vi "GetImages.vi"(4 "File type":T1, 5 "Disabled":bool, 6 "Background Color":u32(colorbox), 7 "image directory":path, 8 "error in":errorcluster, 11 "Boolean in":refnum<class "Boolean.lvclass">) -> (0 "error out":errorcluster, 3 "Boolean out":refnum<class "Boolean.lvclass">)   [LabVIEW 2014, in "Raspberry Pi Compatible Compiler for LabVIEW.lvlib" / "Boolean.lvclass"]
uses:
  Boolean.lvclass
  Control/ImageTypes.ctl
  GObject/GObject.lvclass/GObject.ctl
  GObject/GObject.lvclass
  Raspberry Pi Compatible Compiler for LabVIEW.lvlib
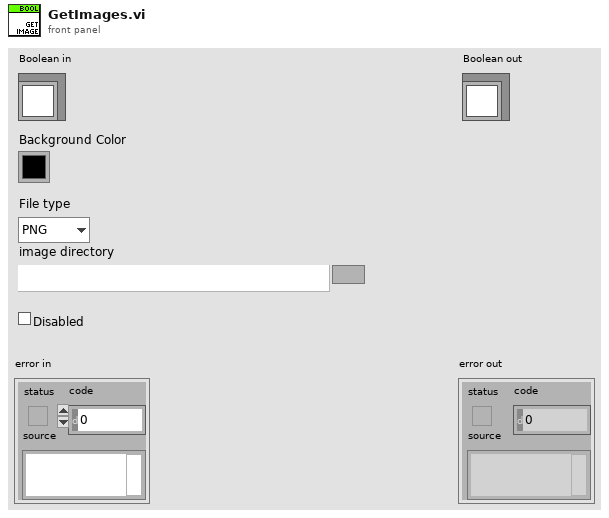
[diagram p1: front panel]
types:
  T1 = typedef "Raspberry Pi Compatible Compiler for LabVIEW.lvlib/ImageTypes.ctl" = enum16{"PNG", "JPEG", "BMP"}
  T2 = enum8{"Enabled", "Disabled", "Disabled and Grayed Out"}
  T3 = enum32{"Invalid", "Standard", "Closed", "Hidden", "Minimized", "Maximized"}
  T4 = typedef "LVPositionTypeDef.ctl" = cluster{"Left":i32, "Top":i32}
  T5 = typedef "imagedata.ctl" = cluster{"image type":i32, "image depth":i32, "image":u8[], "mask":u8[], "colors":u32[], "Rectangle":cluster{"left":i16, "top":i16, "right":i16, "bottom":i16}}
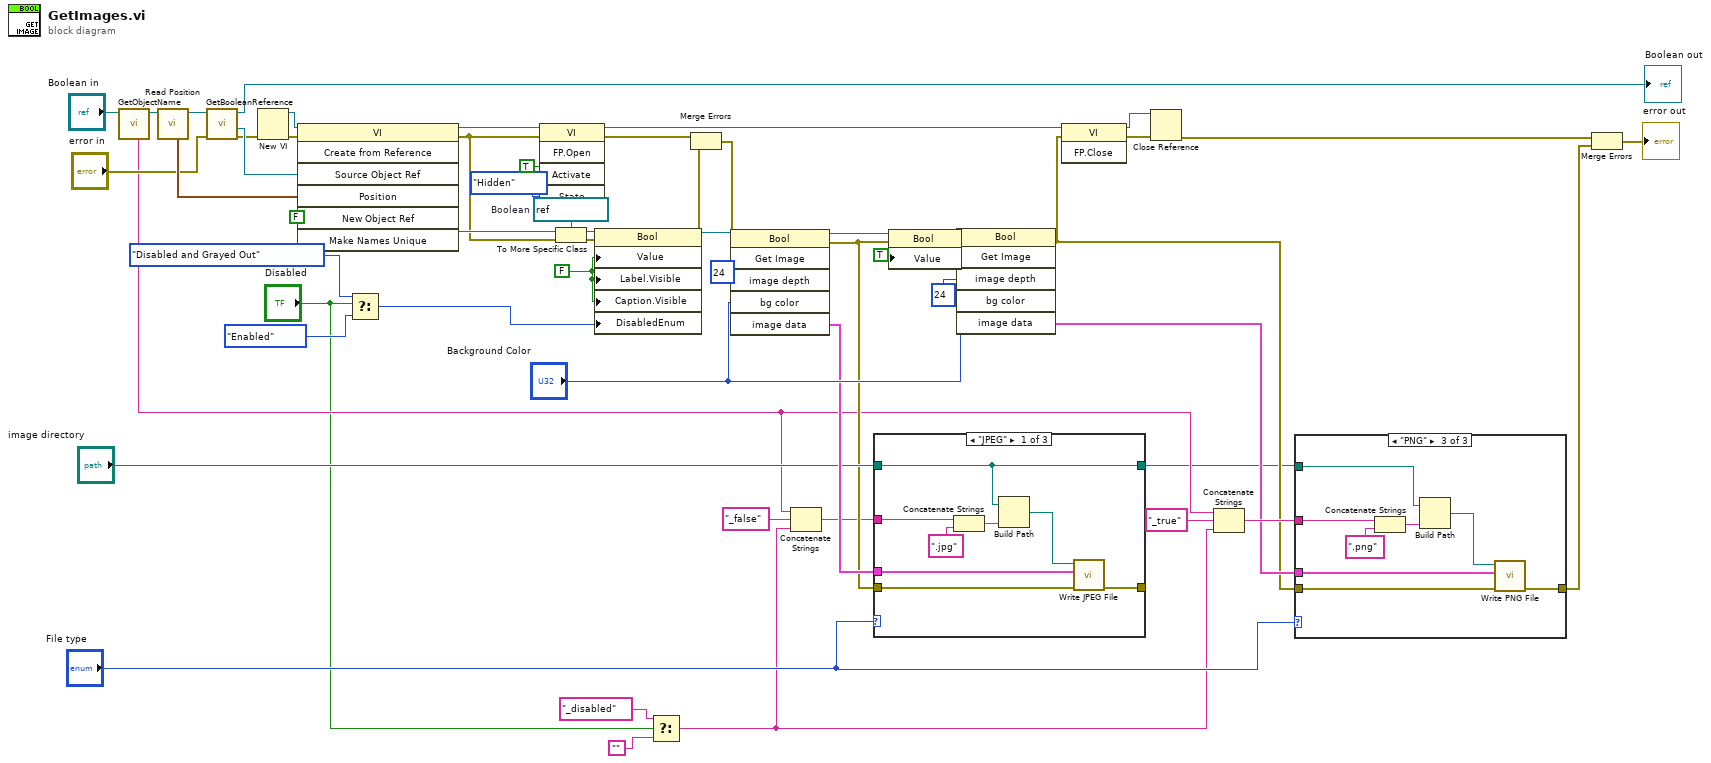
[diagram p0: block diagram]
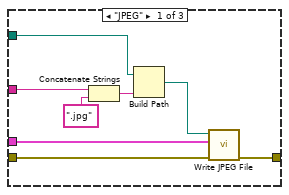
[diagram p2: hidden frame]
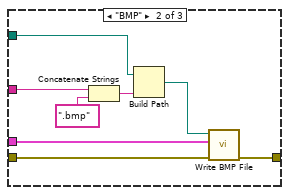
[diagram p3: hidden frame]
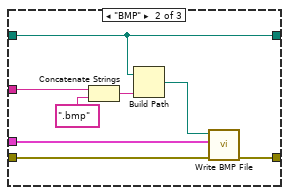
[diagram p4: hidden frame]
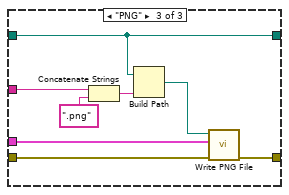
[diagram p5: hidden frame]
diagram:
  w43 = FALSE ("Label.Visible")
  w46 = refnum<vi> refnum  # Boolean
  n1 = call-dynamic "GetObjectName.vi"("GObject in"="Boolean in") -> ("GObject out"=w22:refnum<class "Boolean.lvclass">, "Name"=w14:string)  [unwired: 6 in, 1 out]
  n2 = call "Read Position.vi"("GObject in"=w22) -> ("GObject out"=w29:refnum<class "Boolean.lvclass">, "Position"=w51:T4)  [unwired: 7 in]
  n3 = call "GetBooleanReference.vi"("error in"="error in", "Boolean in"=w29) -> ("error out"=w30:errorcluster, "Boolean reference"=w50:refnum<vi>, "Boolean out"=→"Boolean out":refnum<class "Boolean.lvclass">)  [unwired: 7 in]
  n4 = New VI(8:w30) -> (0:w55:errorcluster, 3:w56:refnum<vi>)  [unwired: 6 in]
  n5 = invoke class="VI" method="Create from Reference"(reference=w56, error in=w55, "Source Object Ref"=w50, "Position"=w51, "Make Names Unique"=FALSE ("Make Names Unique (F)")) -> (reference out=w54:refnum<vi>, error out=w47:errorcluster, "New Object Ref"=w48:refnum<vi>)  [unwired: 2 in, 4 out]
  n6 = Select(t=T2."Disabled and Grayed Out" ("Disabled"), s="Disabled", f=T2."Enabled" ("Disabled")) -> (s? t:f=w5:T2)
  n7 = invoke class="VI" method="FP.Open"(reference=w54, error in=w47, "Activate"=TRUE ("Activate?"), "State"=T3."Hidden") -> (reference out=w33:refnum<vi>, error out=w32:errorcluster)  [unwired: 1 in, 3 out]
  n8 = To More Specific Class(target class=w46, reference=w48, error in=w47) -> (specific class reference=w37:refnum<vi>, error out=w36:errorcluster)
  n9 = property class="Bool"(reference=w37, error in=w36, "Value"=w43, "Label.Visible"=w43, "Caption.Visible"=w43, "DisabledEnum"=w5) -> (reference out=w45:refnum<vi>, error out=w24:errorcluster)
  n10 = Select(t="_disabled" ("string"), s="Disabled", f="") -> (s? t:f=w1:string)
  n11 = Merge Errors(w32, w24) -> (w31:errorcluster)
  n12 = invoke class="Bool" method="Get Image"(reference=w45, error in=w31, "image depth"=24 ("Image Depth"), "bg color"="Background Color") -> (reference out=w42:refnum<vi>, error out=w23:errorcluster, "image data"=w26:T5)  [unwired: 2 in, 3 out]
  n13 = Concatenate Strings(w14, "_false" ("string"), w1) -> (w20:string)
  n14 = case shown="\"JPEG\"" "File type" {
    tunnel: w26 -> [w64 w72 w80]
    tunnel: [w63 w71 w79] -> _
    tunnel: w23 -> [w62 w70 w78]
    tunnel: w20 -> [w61 w69 w77]
    tunnel: "image directory" -> [w57 w65 w73]
    tunnel: [w57 w65 w73] -> w12
    frame "JPEG" {
      n15 = Concatenate Strings(w61, ".jpg" ("string")) -> (w59:string)
      n16 = Build Path(base path=w57, name or relative path=w59) -> (appended path=w58:path)
      n17 = call <vilib>:"Write JPEG File.vi"("error in (no error)"=w62, "image data"=w64, "path to JPEG file"=w58) -> ("error out"=w63:errorcluster)  [unwired: 7 in, 1 out]
    }
    frame "BMP" {
      n18 = Concatenate Strings(w69, ".bmp" ("string")) -> (w67:string)
      n19 = Build Path(base path=w65, name or relative path=w67) -> (appended path=w66:path)
      n20 = call <vilib>:"Write BMP File.vi"("error in (no error)"=w70, "image data"=w72, "path to BMP file"=w66) -> ("error out"=w71:errorcluster)  [unwired: 7 in, 1 out]
    }
    frame "PNG" {
      n21 = Concatenate Strings(w77, ".png" ("string")) -> (w75:string)
      n22 = Build Path(base path=w73, name or relative path=w75) -> (appended path=w74:path)
      n23 = call <vilib>:"Write PNG File.vi"("error in (no error)"=w78, "image data"=w80, "path to PNG file"=w74) -> ("error out"=w79:errorcluster)  [unwired: 7 in, 1 out]
    }
  }
  n24 = property class="Bool"(reference=w42, error in=w23, "Value"=TRUE) -> (reference out=w40:refnum<vi>, error out=w39:errorcluster)
  n25 = invoke class="Bool" method="Get Image"(reference=w40, error in=w39, "image depth"=24 ("Image Depth"), "bg color"="Background Color") -> (error out=w15:errorcluster, "image data"=w16:T5)  [unwired: 2 in, 4 out]
  n26 = invoke class="VI" method="FP.Close"(reference=w33, error in=w15) -> (reference out=w35:refnum<vi>, error out=w34:errorcluster)  [unwired: 1 in, 1 out]
  n27 = Close Reference(reference=w35, error in (no error)=w34) -> (error out=w11:errorcluster)
  n28 = Concatenate Strings(w14, "_true" ("string"), w1) -> (w17:string)
  n29 = case shown="\"PNG\"" "File type" {
    tunnel: w16 -> [w88 w96 w104]
    tunnel: [w87 w95 w103] -> w10
    tunnel: w15 -> [w86 w94 w102]
    tunnel: w17 -> [w85 w93 w101]
    tunnel: w12 -> [w81 w89 w97]
    frame "JPEG" {
      n30 = Concatenate Strings(w85, ".jpg" ("string")) -> (w83:string)
      n31 = Build Path(base path=w81, name or relative path=w83) -> (appended path=w82:path)
      n32 = call <vilib>:"Write JPEG File.vi"("error in (no error)"=w86, "image data"=w88, "path to JPEG file"=w82) -> ("error out"=w87:errorcluster)  [unwired: 7 in, 1 out]
    }
    frame "BMP" {
      n33 = Concatenate Strings(w93, ".bmp" ("string")) -> (w91:string)
      n34 = Build Path(base path=w89, name or relative path=w91) -> (appended path=w90:path)
      n35 = call <vilib>:"Write BMP File.vi"("error in (no error)"=w94, "image data"=w96, "path to BMP file"=w90) -> ("error out"=w95:errorcluster)  [unwired: 7 in, 1 out]
    }
    frame "PNG" {
      n36 = Concatenate Strings(w101, ".png" ("string")) -> (w99:string)
      n37 = Build Path(base path=w97, name or relative path=w99) -> (appended path=w98:path)
      n38 = call <vilib>:"Write PNG File.vi"("error in (no error)"=w102, "image data"=w104, "path to PNG file"=w98) -> ("error out"=w103:errorcluster)  [unwired: 7 in, 1 out]
    }
  }
  n39 = Merge Errors(w11, w10) -> (→"error out":errorcluster)
